vi "Write Handle.vi"(8 "error in (no error)":errorcluster, 11 "Channel in":refnum<class "Channel.lvclass">) -> (0 "error out":errorcluster, 3 "Channel out":refnum<class "Channel.lvclass">)   [LabVIEW 2018, in "Channel.lvclass"]
uses:
  Channel.lvclass
  Channel.lvclass/Channel.ctl
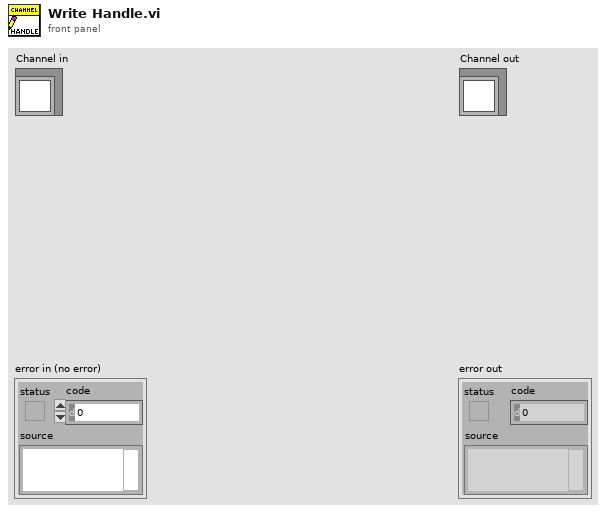
[diagram p1: front panel]
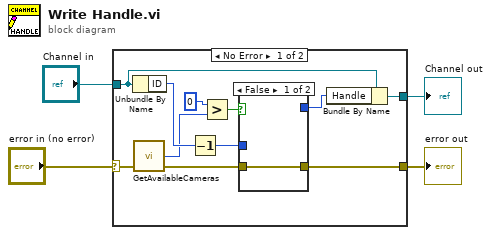
[diagram p0: block diagram]
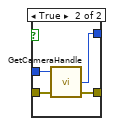
[diagram p2: hidden frame]
diagram:
  n1 = case shown="No Error" "error in (no error)" {
    selector: "error in (no error)" -> [w8 w21]
    tunnel: [w14 w21] -> w3
    tunnel: [w15 w22] -> w1
    tunnel: "Channel in" -> [w12 w22]
    frame No Error {
      n2 = Unbundle By Name(w12) -> ("ID"=w11:u8)
      n3 = call <userlib>:"GetAvailableCameras.vi"("error in (no error)"=w8) -> ("error out"=w9:errorcluster, "totalCameras"=w7:i32)  [unwired: 2 in, 1 out]
      n4 = Decrement(x=w11) -> (x-1=w10:u8)
      n5 = Greater?(x=0, y=w7) -> (0:w5:bool)
      n6 = case shown="False" w5 {
        tunnel: [w16 w20] -> w14
        tunnel: [_ w19] -> w13
        tunnel: w10 -> [_ w18]
        tunnel: w9 -> [w16 w17]
        frame False {
        }
        frame True {
          n7 = call <userlib>:"GetCameraHandle.vi"("error in (no error)"=w17, "cameraIndex"=w18) -> ("error out"=w20:errorcluster, "cameraHandle"=w19:i32)  [unwired: 1 in, 1 out]
        }
      }
      n8 = Bundle By Name(cluster=w12, "Handle"=w13) -> (w15:refnum<class "Channel.lvclass">)
    }
    frame Error {
    }
  }
  "error out" <- w3
  "Channel out" <- w1
